vi "T_control.vi"(0 "Ref vel":dbl=1.0, 1 "VS_CAN":dbl, 7 "pid gain":dbl[](array[numeric])) -> (14 "Ref APS":dbl)   [LabVIEW 2015]
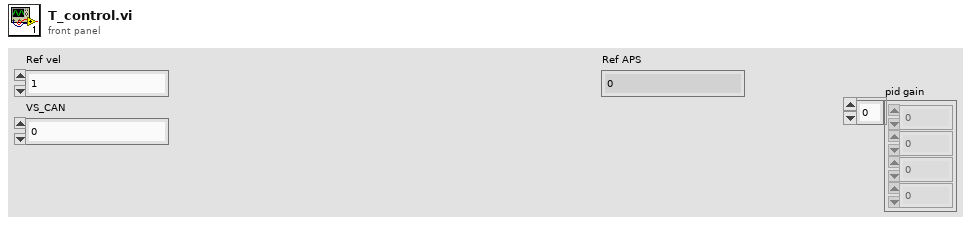
[diagram p1: front panel]
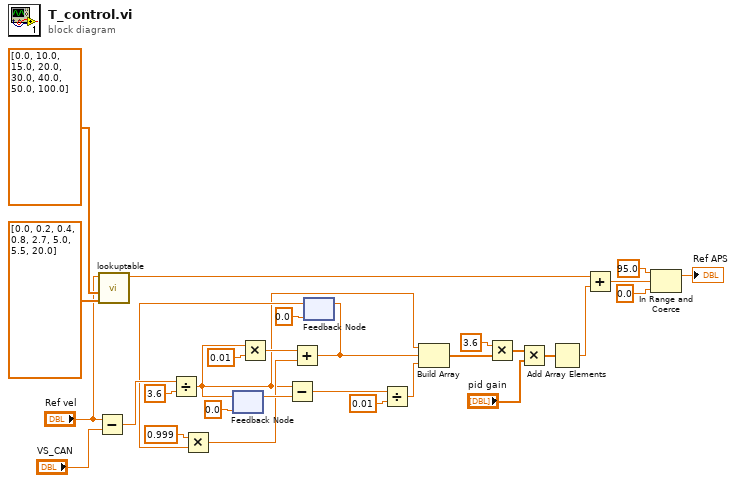
[diagram p0: block diagram]
diagram:
  n1 = Subtract(x="Ref vel", y="VS_CAN") -> (x-y=w30:dbl)
  n2 = call "lookuptable.vi"("array_y"=dbl[] [0.0, 0.2, 0.4, 0.8, 2.7, 5.0, 5.5, 20.0] ("array_x"), "array_x"=dbl[] [0.0, 10.0, 15.0, 20.0, 30.0, 40.0, 50.0, 100.0], "x"="Ref vel") -> ("y"=w26:dbl)  [unwired: 8 in]
  n3 = Divide(x=w30, y=3.6) -> (x/y=w6:dbl)
  n4 = feedback #1(0.0) -> (w21:dbl)
  n5 = feedback-in #1(w6) -> ()
  n6 = Multiply(x=w6, y=0.01) -> (x*y=w17:dbl)
  n7 = Subtract(x=w6, y=w21) -> (x-y=w20:dbl)
  n8 = feedback #2(0.0) -> (w14:dbl)
  n9 = Multiply(x=0.999, y=w14) -> (x*y=w13:dbl)
  n10 = Add(x=w17, y=w13) -> (x+y=w9:dbl)
  n11 = feedback-in #2(w9) -> ()
  n12 = Divide(x=w20, y=0.01) -> (x/y=w8:dbl)
  n13 = Build Array(w6, w9, w8) -> (w4:dbl[])
  n14 = Multiply(x=3.6 ("y"), y=w4) -> (x*y=w3:dbl[])
  n15 = Multiply(x=w3, y="pid gain") -> (x*y=w15:dbl[])
  n16 = Add Array Elements(numeric array=w15) -> (sum=w27:dbl)
  n17 = Add(x=w26, y=w27) -> (x+y=w25:dbl)
  n18 = In Range and Coerce(upper limit=95.0 ("x+y"), x=w25, lower limit=0.0) -> (coerced(x)=→"Ref APS":dbl)  [unwired: 1 out]
